vi "HRM-close-main.vi"(8 "error in (no error)":errorcluster, 11 "init cluster":T1) -> (0 "error out":errorcluster)   [LabVIEW 2020]
uses:
  HRM-init-cluster.ctl
  HRM-init-user_events.ctl
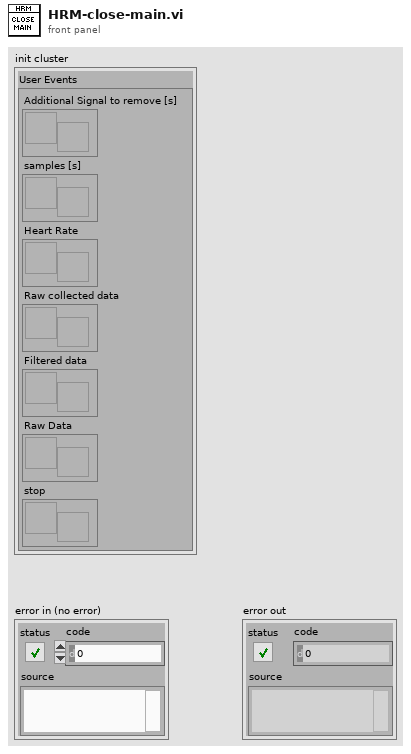
[diagram p1: front panel]
types:
  T1 = typedef "HRM-init-cluster.ctl" = cluster{"User Events":T2}
  T2 = typedef "HRM-init-user_events.ctl" = cluster{"Additional Signal to remove [s]":refnum<user-event>, "samples [s]":refnum<user-event>, "Heart Rate":refnum<user-event>, "Raw collected data":refnum<user-event>, "Filtered data":refnum<user-event>, "Raw Data":refnum<user-event>, "stop":refnum<user-event>}
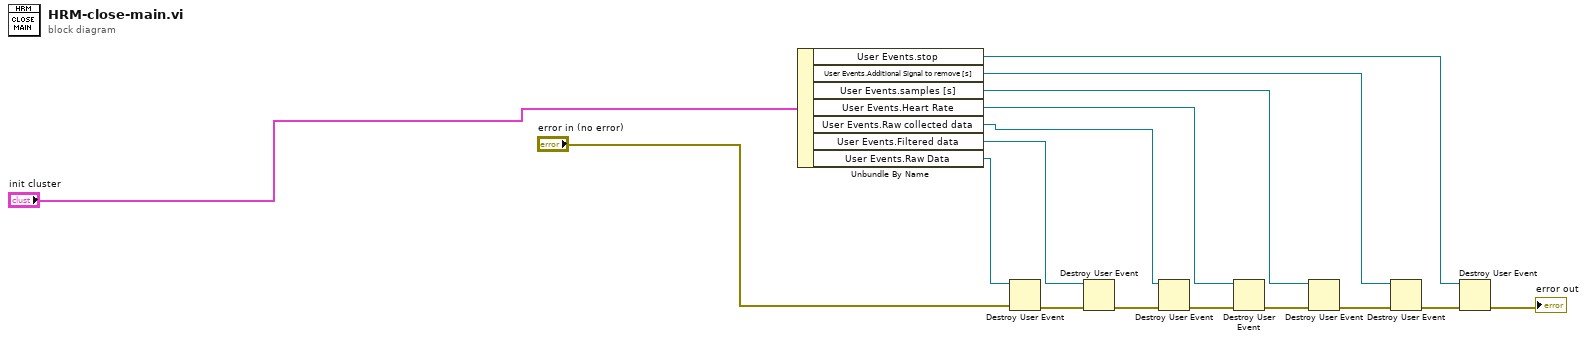
[diagram p0: block diagram]
diagram:
  n1 = Unbundle By Name("init cluster") -> ("User Events.stop"=w13:refnum<user-event>, "User Events.Additional Signal to remove [s]"=w6:refnum<user-event>, "User Events.samples [s]"=w5:refnum<user-event>, "User Events.Heart Rate"=w4:refnum<user-event>, "User Events.Raw collected data"=w3:refnum<user-event>, "User Events.Filtered data"=w2:refnum<user-event>, "User Events.Raw Data"=w1:refnum<user-event>)
  n2 = Destroy User Event(user event=w1, error in="error in (no error)") -> (error out=w7:errorcluster)
  n3 = Destroy User Event(user event=w2, error in=w7) -> (error out=w8:errorcluster)
  n4 = Destroy User Event(user event=w3, error in=w8) -> (error out=w9:errorcluster)
  n5 = Destroy User Event(user event=w4, error in=w9) -> (error out=w10:errorcluster)
  n6 = Destroy User Event(user event=w5, error in=w10) -> (error out=w11:errorcluster)
  n7 = Destroy User Event(user event=w6, error in=w11) -> (error out=w12:errorcluster)
  n8 = Destroy User Event(user event=w13, error in=w12) -> (error out=→"error out":errorcluster)
